vi "MessageOut_Communication.vi"(8 "Error In":errorcluster, 11 "Spaceship in":refnum<class "Spaceship.lvclass">) -> (0 "Error Out":errorcluster, 2 "Message Out":string, 3 "Spaceship out":refnum<class "Spaceship.lvclass">)   [LabVIEW 2021, in "Spaceship.lvclass"]
doc: "Preview string message in class objet queue."
uses:
  Spaceship.lvclass
  Spaceship.lvclass/Spaceship.ctl
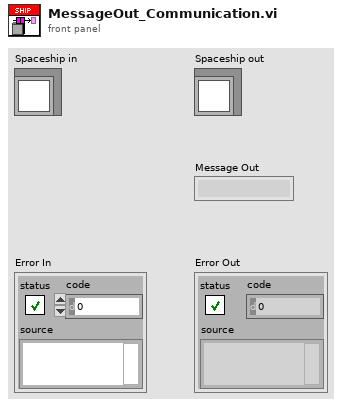
[diagram p1: front panel]
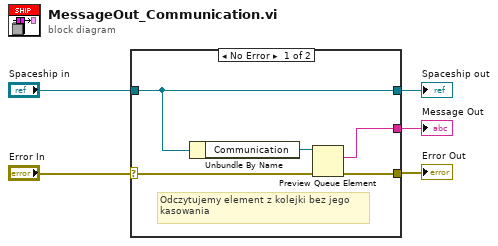
[diagram p0: block diagram]
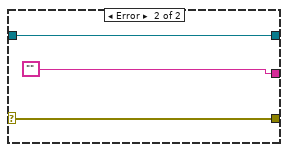
[diagram p2: hidden frame]
diagram:
  n1 = case shown="No Error" "Error In" {
    selector: "Error In" -> [w9 w13]
    tunnel: [w7 w13] -> w4
    tunnel: [w10 w12] -> w2
    tunnel: "Spaceship in" -> [w10 w12]
    tunnel: [w6 ""] -> w1
    frame No Error {
      # "Odczytujemy element z kolejki bez jego\nkasowania"
      n2 = Unbundle By Name(w10) -> ("Communication"=w8:refnum<queue>)
      n3 = Preview Queue Element(queue=w8, error in (no error)=w9) -> (element=w6:string, error out=w7:errorcluster)  [unwired: 1 in, 2 out]
    }
    frame Error {
    }
  }
  "Error Out" <- w4
  "Spaceship out" <- w2
  "Message Out" <- w1
